vi "Main_Andor_Multi_SI_ver1.vi"() -> ()   [LabVIEW 2014]
doc: "This is the main user interface of the Raman spectroscopy system."
uses:
  <userlib>/atmcd64d.llb/AcquisitionMode_mode typedef.ctl
  <userlib>/atmcd64d.llb/ReadMode_mode typedef.ctl
  <userlib>/atmcd64d.llb/Shutter_mode typedef.ctl
  <userlib>/atmcd64d.llb/Shutter_type typedef.ctl
  <userlib>/atmcd64d.llb/TriggerMode_mode typedef.ctl
  TypeDef/GalvoInput.ctl
  <userlib>/atmcd64d.llb/Error Code Enum typedef.ctl
  TypeDef/States.ctl
panel:
  in  "Tab Control":enum32{"Main", "Andor", "Galvo"}(tab)
  in  "Pause":bool
  in  "Scan Range":T1={"Ver_V/H"=0.35, "Hor_V/W"=0.35, "Ver_r"=5.0, "Hor_r"=5.0}
  in  "Scan Resolusion":T2={"Ver_V"=0.35, "Hor_H"=0.35, "Ver_Pix"=214.0, "Hor_Pix"=200.0}
  in  "Galvo Center":bool
  out "Galvo":bool
  out "Spot Y":dbl
  out "Spot X":dbl
  in  "Quit":bool
  out "Initialization finished":bool
  in  "Galvo Stop":bool
  in  "Galvo Scan":bool
  out "Andor":bool
  out "CurrentFrame":i32
  in  "Set":bool
  in  "AndorSnap":bool
  out "SaveStatus":bool
  in  "FilePath":string="C:\\Users\\light\\Desktop\\Data"
  in  "Exit":bool
  out "ShutDown":cluster{"CoolOff":bool, "ShutDown":bool}
  in  "Mode":T8={"AcqMode"=enum."Single Scan", "ReadMode"=enum."Single-Track", "ShutterMode"=enum."Auto", "GateMode"=enum."TTL High", "TriggerMode"=enum."Internal"}
  in  "AcqSet":T9={"openingtime"=0, "closingtime/ms"=0, "ExposureTime/s"=0.1, "AccumCycTime"=0.0, "AccumCycNum"=1, "KineticNum"=1, "KineticTime"=0.0} {"KineticTime" format="%.5f"; "AccumCycNum" format="%.5f"; "AccumCycTime" format="%.5f"; "ExposureTime/s" format="%.5f"; "closingtime/ms" format="%.2f"; "openingtime" format="%.2f"}
  out "Timing":T10 {"kinetic" format="%.7f"; "accumulate" format="%.7f"; "exposure" format="%.7f"}
  out "SetOut":T11
  in  "MultiTrack":cluster{"StartRow":i32, "EndRow":i32}={"StartRow"=131, "EndRow"=143}
  out "SetStatus":bool
  out "CurrentTemp":i32
  out "DevInit":bool
  out "DevSize":cluster{"xpixels":i32, "ypixels":i32}
  out "HardWVersion":T12
  out "SoftWVersion":T13
  out "Speeds":T14
  in  "TargetTemp":i32
  out "CoolerON":T15
  out "GetStatus":T16
  in  "YOffset":dbl=8.2 caption="Offset"
  in  "XOffset":dbl=4.0 caption="Offset"
  out "Sample Rate":dbl=1000.0 format="%0.2f"
  out "Waveform Graph":waveform(dbl)[](graph)=[{"t0"=timestamp(0 s since 1904-01-01), "dt"=0.001, "Y"=[]}]
  in  "ZOffset":dbl caption="Offset"
  in  "Galvo":T17={"Sample Rate"=1000.0, "Sample Clock Source"="OnboardClock", "Max Voltage"=10.0, "Min Voltage"=-10.0, "Physical Channel(s)"="Dev1/ao0,Dev1/ao1,Dev1/ao3"}
  # "Objective: CFI Plan Fluor ELWD 60x (1.27 NA) \nThe depth of field: 1.78 um\nPixel Size: 0.0877um/px"
  # "Kinetics->SignleTrack"
  # "Galvo Control"
  # "50Hz->1s"
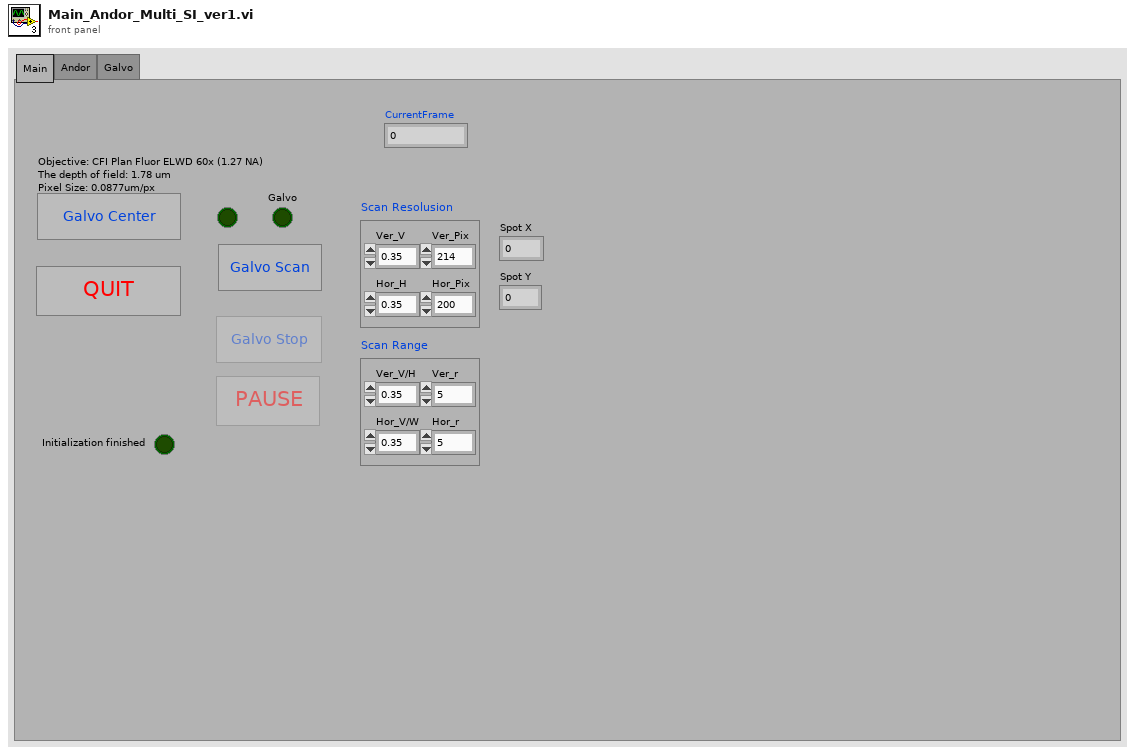
[diagram p1: front panel]
types:
  T1 = cluster{"Ver_V/H":dbl, "Hor_V/W":dbl, "Ver_r":dbl, "Hor_r":dbl}
  T2 = cluster{"Ver_V":dbl, "Hor_H":dbl, "Ver_Pix":dbl, "Hor_Pix":dbl}
  T3 = typedef "AcquisitionMode_mode typedef.ctl" = enum16{"Reserved (0)", "Single Scan", "Accumulate", "Kinetics", "Fast Kinetics", "Run Till Abort", "Reserved (6)", "Reserved (7)", "Reserved (8)", "Time Delayed Integration"}
  T4 = typedef "ReadMode_mode typedef.ctl" = enum16{"Full Vertical Binning", "Multi-Track", "Random-Track", "Single-Track", "Image"}
  T5 = typedef "Shutter_mode typedef.ctl" = enum16{"Auto", "Open", "Close", "N/A (3)", "Open FVB Series", "Open Any Series"}
  T6 = typedef "Shutter_type typedef.ctl" = enum16{"TTL Low", "TTL High"}
  T7 = typedef "TriggerMode_mode typedef.ctl" = enum16{"Internal", "External", "N/A (2)", "N/A (3)", "N/A (4)", "N/A (5)", "External Start", "External Exposure (Bulb)", "N/A (8)", "External FVB EM", "Software", "N/A (11)", "External Charge Shifting"}
  T8 = cluster{"AcqMode":T3, "ReadMode":T4, "ShutterMode":T5, "GateMode":T6, "TriggerMode":T7}
  T9 = cluster{"openingtime":i32, "closingtime/ms":i32, "ExposureTime/s":sgl, "AccumCycTime":sgl, "AccumCycNum":i32, "KineticNum":i32, "KineticTime":sgl}
  T10 = cluster{"exposure":sgl, "accumulate":sgl, "kinetic":sgl}
  T11 = cluster{"Height":i32, "Width":i32, "bottom":i32, "gap":i32}
  T12 = cluster{"PCB":u32, "Flex":u32, "dummy1":u32, "dummy2":u32, "dummy3":u32, "dummy4":u32}
  T13 = cluster{"eprom":u32, "cofFile":u32, "vxdRev":u32, "vxdVer":u32, "dllRev":u32, "dllVer":u32}
  T14 = cluster{"NVS":i32, "VS":i32, "NHS":dbl, "HS":i32}
  T15 = cluster{"SetTemp":bool, "CoolerOn":bool, "Stablized":bool}
  T16 = cluster{"GetDetector":bool, "GetHardVer":bool, "GetNVS":bool, "GetVS":bool, "GetSotfVer":bool, "GetNHS":bool, "GetHS":bool}
  T17 = typedef "GalvoInput.ctl" = cluster{"Sample Rate":dbl, "Sample Clock Source":tag, "Max Voltage":dbl, "Min Voltage":dbl, "Physical Channel(s)":tag}
  T18 = typedef "States.ctl" = enum16{"Initialize", "CMOS live", "Shut down"}
  T19 = enum8{"Enabled", "Disabled", "Disabled and Grayed Out"}
  T20 = typedef "Error Code Enum typedef.ctl" = enum32{"N/A (0)", "DRV_ERROR_CODES", "DRV_SUCCESS", "DRV_VXDNOTINSTALLED", "DRV_ERROR_SCAN", "DRV_ERROR_CHECK_SUM", "DRV_ERROR_FILELOAD", "DRV_UNKNOWN_FUNC", "DRV_ERROR_VXD_INIT", "DRV_ERROR_ADDRESS", "DRV_ERROR_PAGELOCK", "DRV_ERROR_PAGEUNLOCK", "DRV_ERROR_BOARDTEST", "DRV_ERROR_ACK", "DRV_ERROR_UP_FIFO", "DRV_ERROR_PATTERN", "N/A (16)", "DRV_ACQUISITION_ERRORS", "DRV_ACQ_BUFFER", "DRV_ACQ_DOWNFIFO_FULL", "DRV_PROC_UNKONWN_INSTRUCTION", "DRV_ILLEGAL_OP_CODE", "DRV_KINETIC_TIME_NOT_MET", "DRV_ACCUM_TIME_NOT_MET", "DRV_NO_NEW_DATA", "N/A (25)", "DRV_SPOOLERROR", "N/A (27)", "N/A (28)", "N/A (29)", "N/A (30)", "N/A (31)", "N/A (32)", "DRV_TEMPERATURE_CODES", "DRV_TEMPERATURE_OFF", "DRV_TEMPERATURE_NOT_STABILIZED", "DRV_TEMPERATURE_STABILIZED", "DRV_TEMPERATURE_NOT_REACHED", "DRV_TEMPERATURE_OUT_RANGE", "DRV_TEMPERATURE_NOT_SUPPORTED", "DRV_TEMPERATURE_DRIFT", "N/A (41)", "N/A (42)", "N/A (43)", "N/A (44)", "N/A (45)", "N/A (46)", "N/A (47)", "N/A (48)", "DRV_GENERAL_ERRORS", "DRV_INVALID_AUX", "DRV_COF_NOTLOADED", "DRV_FPGAPROG", "DRV_FLEXERROR", "DRV_GPIBERROR", "N/A (55)", "N/A (56)", "N/A (57)", "N/A (58)", "N/A (59)", "N/A (60)", "N/A (61)", "N/A (62)", "N/A (63)", "DRV_DATATYPE", "DRV_DRIVER_ERRORS", "DRV_P1INVALID", "DRV_P2INVALID", "DRV_P3INVALID", "DRV_P4INVALID", "DRV_INIERROR", "DRV_COFERROR", "DRV_ACQUIRING", "DRV_IDLE", "DRV_TEMPCYCLE", "DRV_NOT_INITIALIZED", "DRV_P5INVALID", "DRV_P6INVALID", "DRV_INVALID_MODE", "DRV_INVALID_FILTER", "DRV_I2CERRORS", "DRV_I2CDEVNOTFOUND", "DRV_I2CTIMEOUT", "DRV_P7INVALID", "N/A (84)", "N/A (85)", "N/A (86)", "N/A (87)", "N/A (88)", "N/A (89)", "DRV_IOCERROR", "DRV_VRMVERSIONERROR"}
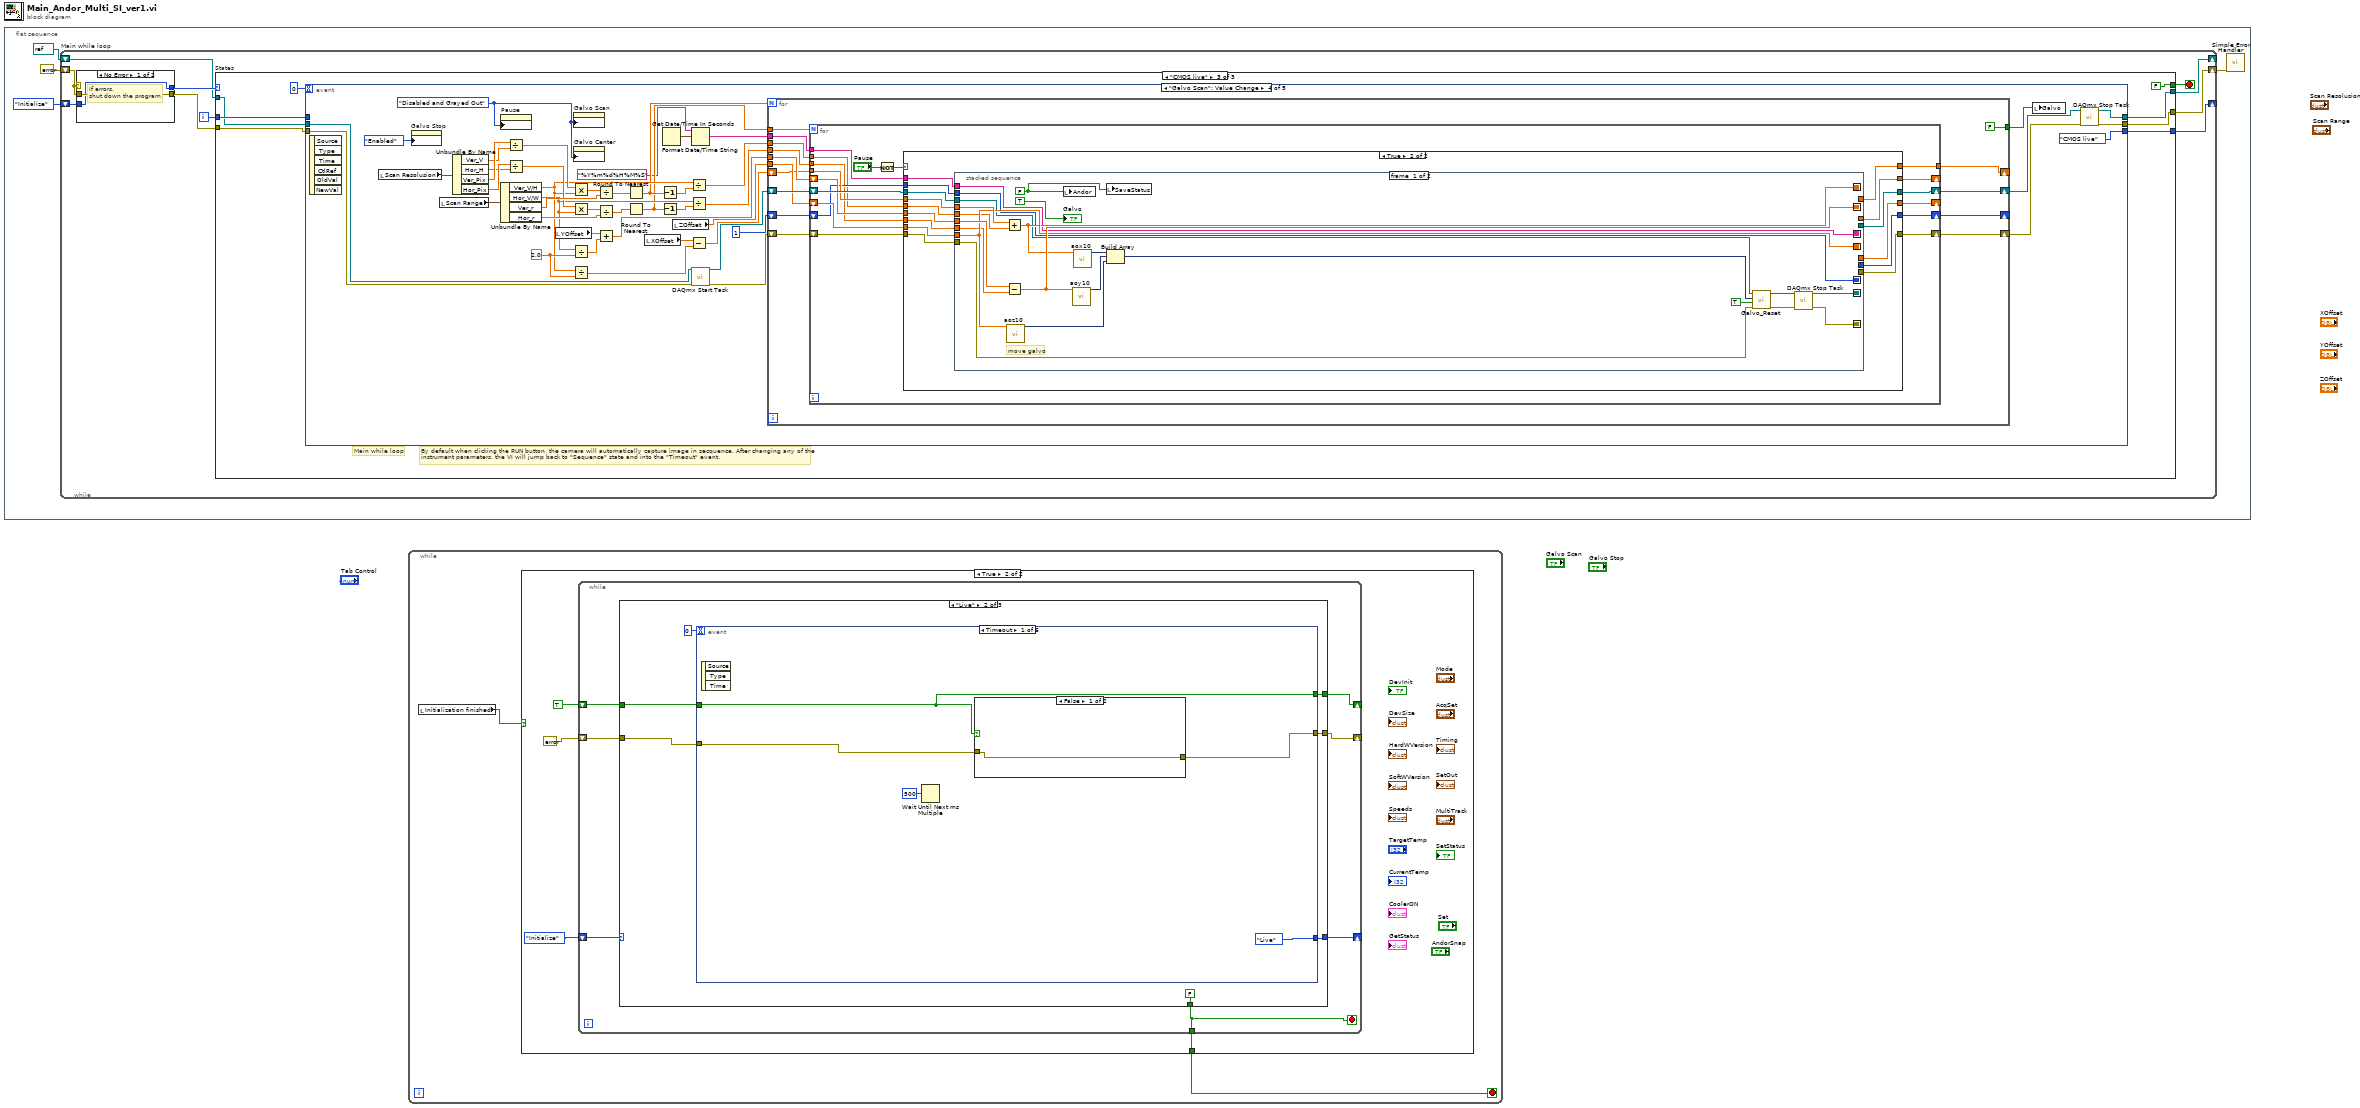
[diagram p0: block diagram]
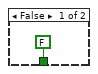
[diagram p2: hidden frame]
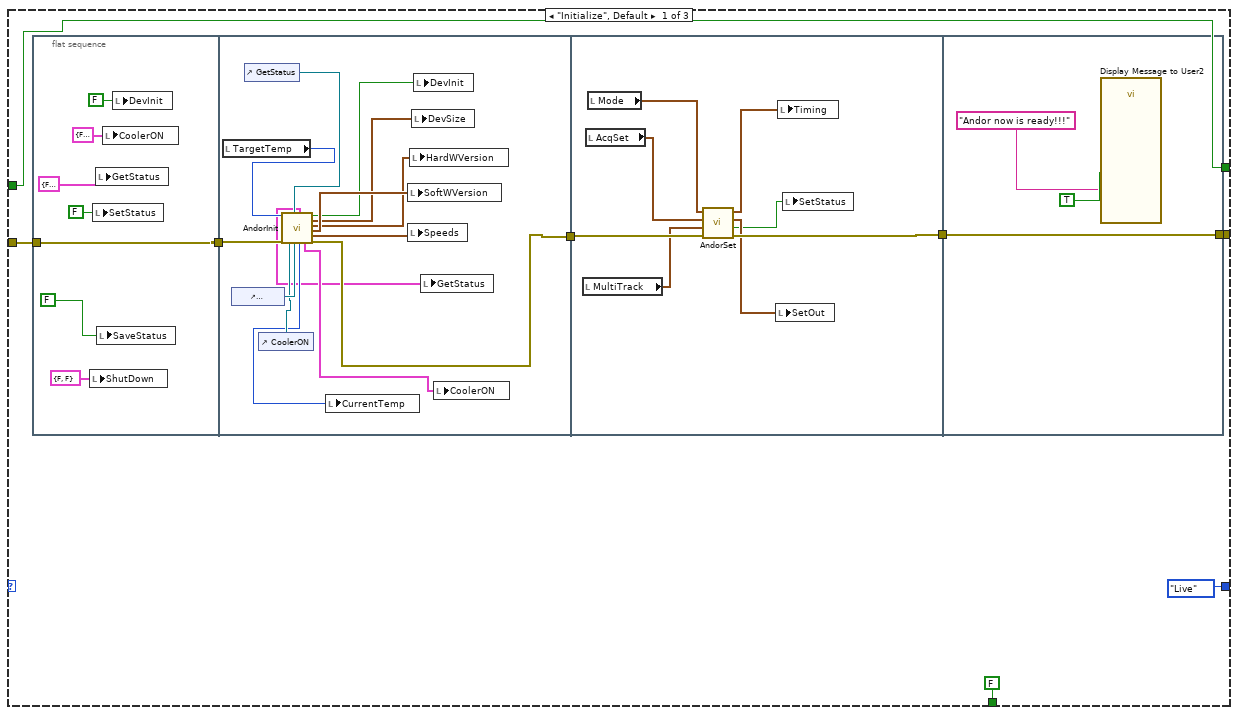
[diagram p3: hidden frame]
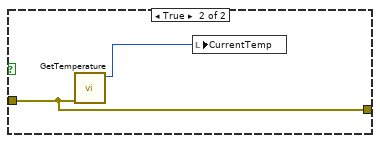
[diagram p4: hidden frame]
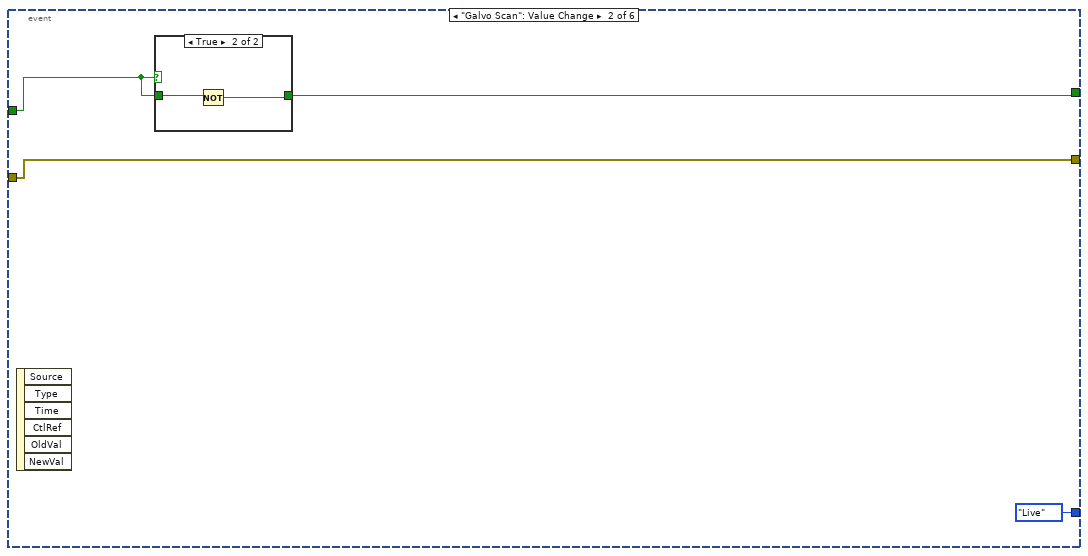
[diagram p5: hidden frame]
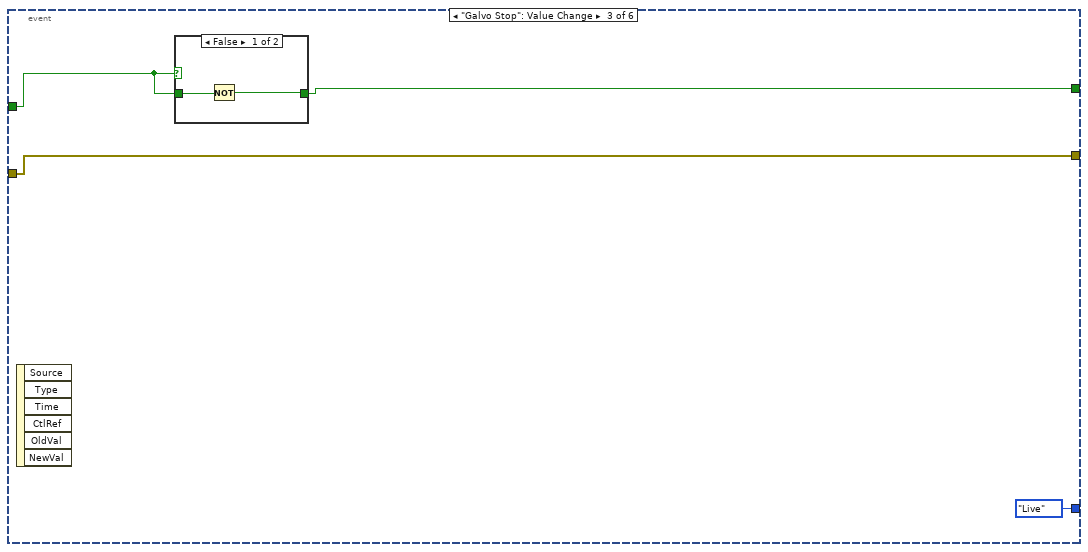
[diagram p7: hidden frame]
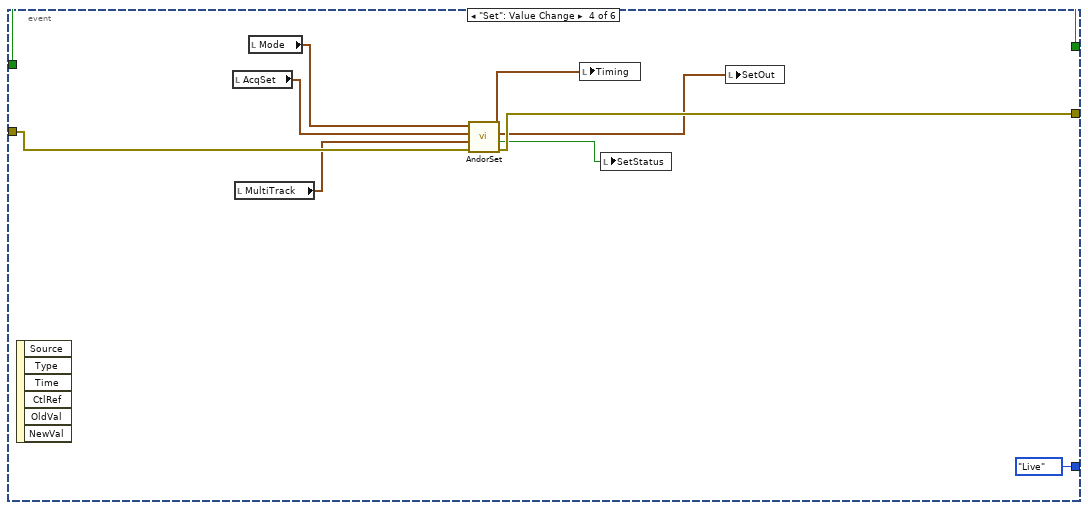
[diagram p9: hidden frame]
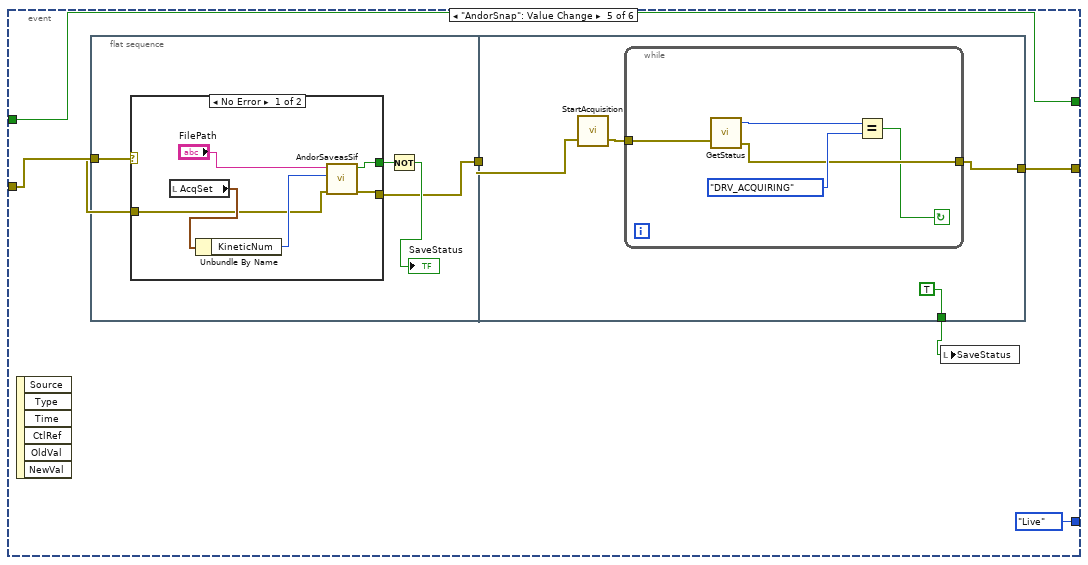
[diagram p10: hidden frame]
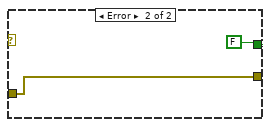
[diagram p11: hidden frame]
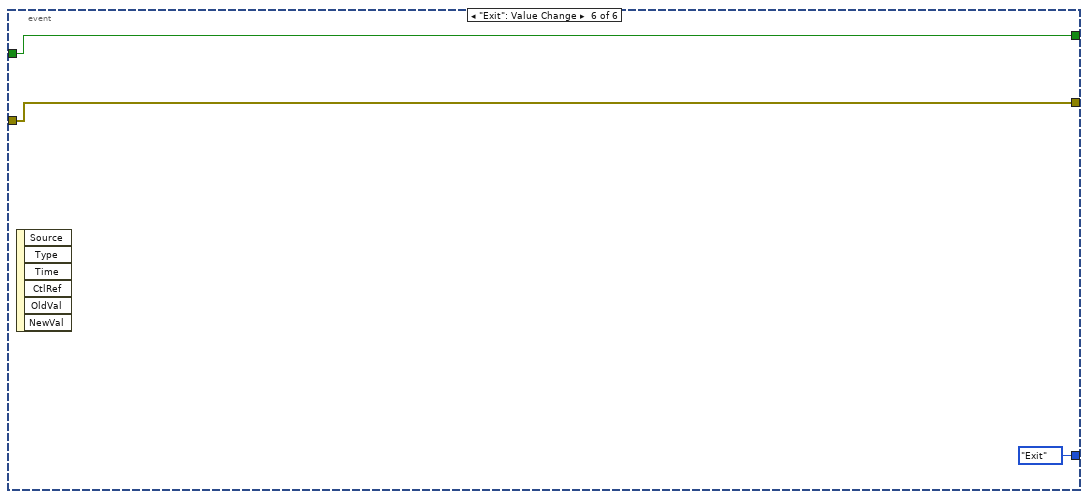
[diagram p12: hidden frame]
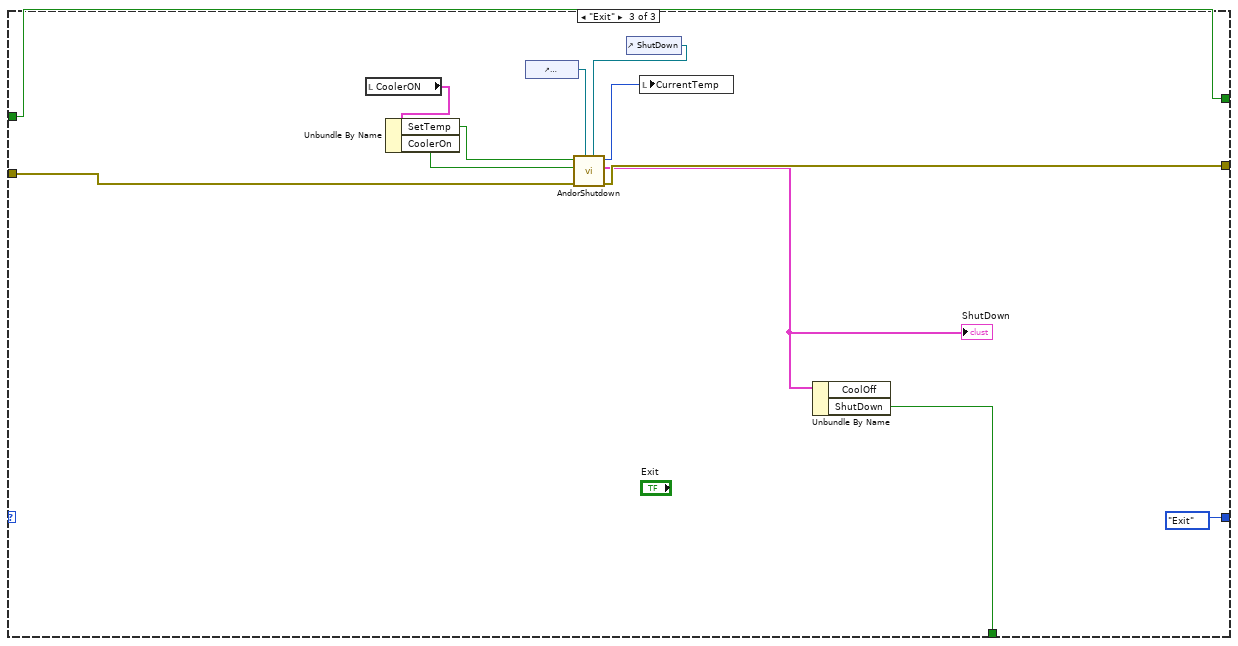
[diagram p13: hidden frame]
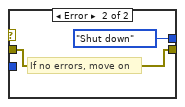
[diagram p14: hidden frame]
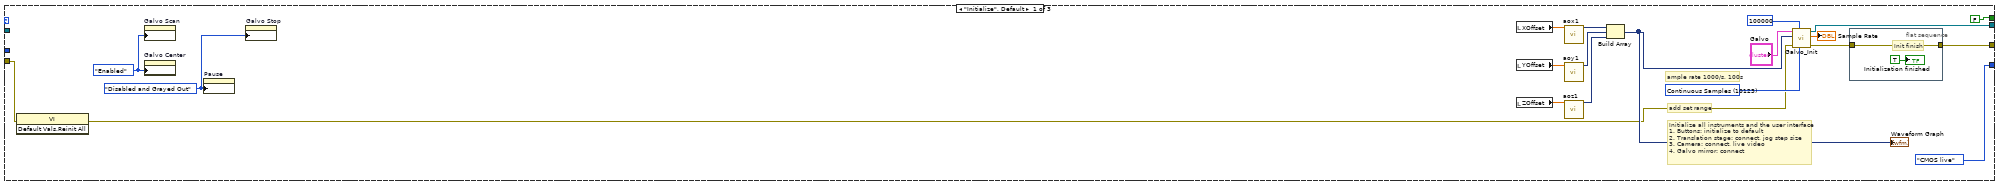
[diagram p15: hidden frame]
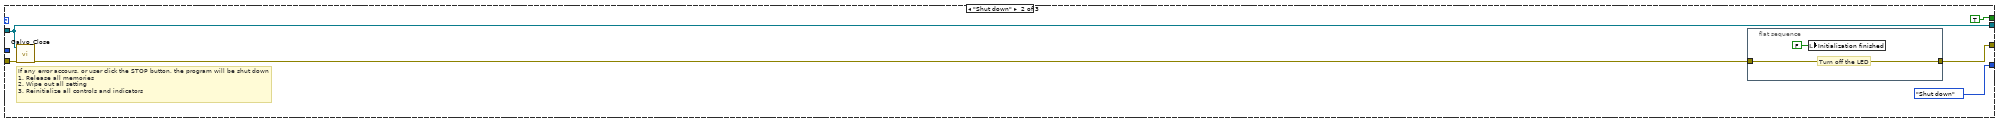
[diagram p16: hidden frame]
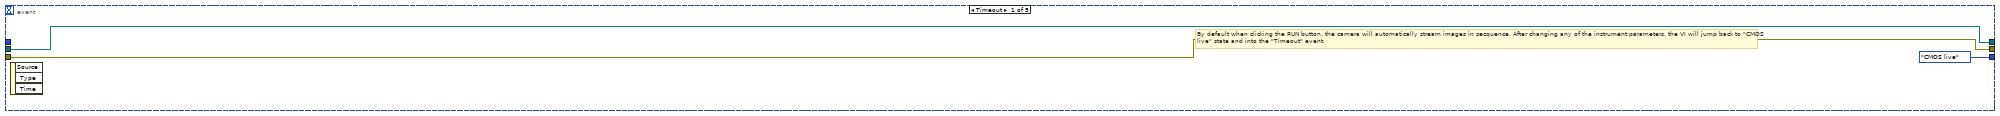
[diagram p17: hidden frame]
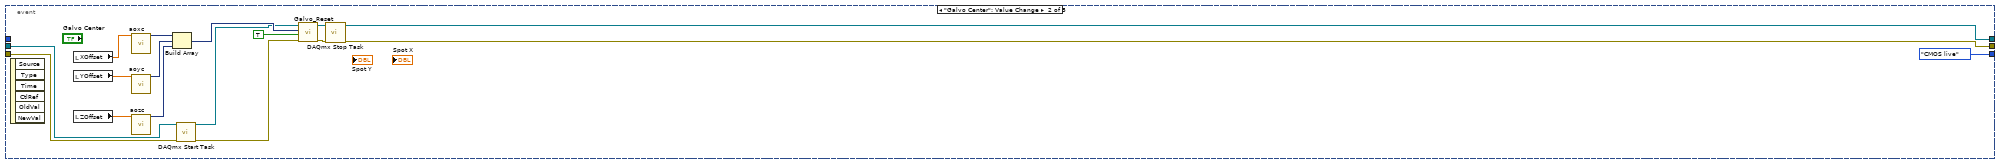
[diagram p18: hidden frame]
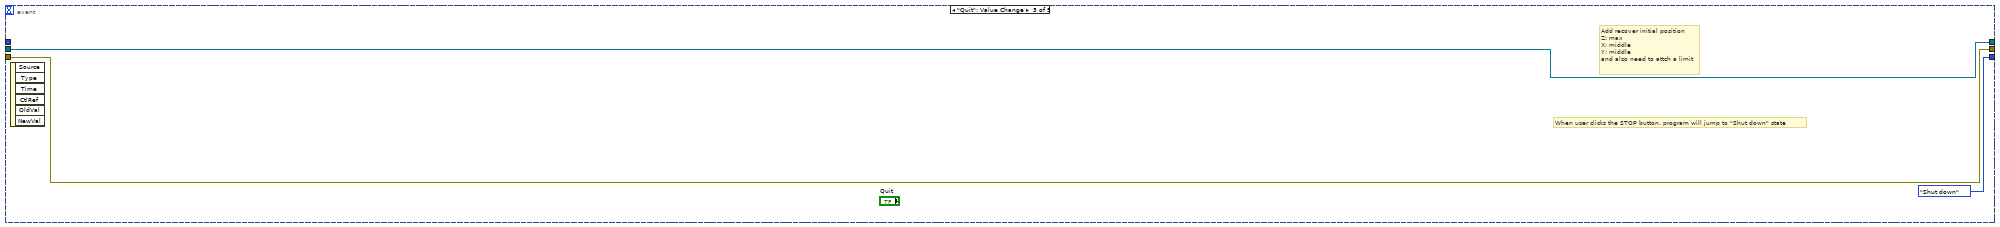
[diagram p19: hidden frame]
diagram:
  n1 = flat-sequence {
    frame #0 {
      n2 = while "Main while loop" {
        shift-right: [w9] -> _
        shift-left: States."Initialize" -> [w14]
        shift-right: [w12] -> w2
        shift-left: errorcluster {"status"=FALSE, "code"=0, "source"=""} ("error out") -> [w8]
        shift-right: [w6] -> _
        shift-left: refnum<k21> refnum ("task out") -> [w5]
        i -> [w7]
        stop <- w10 stop-if-true
        n3 = case shown="No Error" w8 {
          tunnel: w8 -> [w16 w18]
          tunnel: [w16 w18] -> w11
          tunnel: w14 -> [w15 _]
          tunnel: [w15 States."Shut down"] -> w13
          frame No Error {
            # "If errors,\nshut down the program"
          }
          frame Error {
            # "If no errors, move on"
          }
        }
        n4 = case "States" shown="\"CMOS live\"" w13 {
          tunnel: [w36 w41 w54] -> w12
          tunnel: w11 -> [w37 w42 w55]
          tunnel: [FALSE TRUE FALSE] -> w10
          tunnel: [States."CMOS live" States."Shut down" w56] -> w9
          tunnel: w7 -> [_ _ w52]
          tunnel: [w33 w44 w50] -> w6
          tunnel: w5 -> [_ w44 w51]
          frame "Initialize", Default {
            w19 = T19."Disabled and Grayed Out" ("Disabled")
            w22 = T19."Enabled" ("Disabled")
            w28 = 10123 items=["Finite Samples"=10178, "Continuous Samples"=10123, "Hardware Timed Single Point"=12522] ("Sample Mode")
            # "ample rate 1000/s, 100s"
            # "add set range"
            # "Initialize all instruments and the user interface\n1. Buttons: initialize to default\n2. Translation stage: connect, jog step size\n3. Camera: connect, live video\n4. Galvo mirror: connect"
            n5 = invoke class="VI" method="Default Vals.Reinit All"(error in=w37) -> (error out=w21:errorcluster)  [unwired: 2 in, 2 out]
            n6 = property on="Galvo Scan" class="Bool"("DisabledEnum"=w22) -> ()  [unwired: 2 in, 2 out]
            n7 = property on="Galvo Center" class="Bool"("DisabledEnum"=w22) -> ()  [unwired: 2 in, 2 out]
            n8 = property on="Pause" class="Bool"("DisabledEnum"=w19) -> ()  [unwired: 2 in, 2 out]
            n9 = property on="Galvo Stop" class="Bool"("DisabledEnum"=w19) -> ()  [unwired: 2 in, 2 out]
            n10 = local read "XOffset"() -> (w25:dbl)
            n11 = local read "YOffset"() -> (w24:dbl)
            n12 = local read "ZOffset"() -> (w23:dbl)
            n13 = call "aox1"("Offset"=w25) -> ("DC"=w27:dynamicdata)  [unwired: 13 in, 1 out]
            n14 = call "aoy1"("Offset"=w24) -> ("DC"=w26:dynamicdata)  [unwired: 13 in, 1 out]
            n15 = call "aoz1"("Offset"=w23) -> ("DC"=w31:dynamicdata)  [unwired: 13 in, 1 out]
            n16 = Build Array(w27, w26, w31) -> (w30:dynamicdata[])
            "Waveform Graph" <- w30
            n17 = call "Galvo_Init.vi"("Sample Mode"=w28, "samples per channel"=100000, "error in"=w21, "Signal array"=w30, "Galvo_Input"="Galvo") -> ("error out"=w32:errorcluster, "Actual Sample Rate"=→"Sample Rate":dbl, "task out"=w33:refnum<k21>)  [unwired: 4 in]
            n18 = flat-sequence {
              tunnel: w32 -> [w40]
              tunnel: [w40] -> w36
              frame #0 {
                # "Init finish"
                "Initialization finished" <- TRUE ("Initialization finished")
              }
            }
          }
          frame "Shut down" {
            # "If any error accours, or user click the STOP button, the program will be shut down\n1. Release all memories\n2. Wipe out all setting\n3. Reinitialize all controls and indicators"
            n19 = call "Galvo_Close.vi"("error in"=w42, "task/channels in"=w44) -> ("error out"=w43:errorcluster)  [unwired: 9 in]
            n20 = flat-sequence {
              tunnel: w43 -> [w47]
              tunnel: [w47] -> w41
              frame #0 {
                # "Turn off the LED"
                n21 = local write "Initialization finished"(FALSE ("Initialization finished")) -> ()
              }
            }
          }
          frame "CMOS live" {
            # "Main while loop"
            # "By default when clicking the RUN button, the camera will automatically capture image in secquence. After changing any of the \ninstrument parameters, the VI will jump back to \"Sequence\" state and into the \"Timeout\" event."
            n22 = event shown="[3] \"Galvo Scan\": Value Change" {
              selector: _ -> [_ _ _ _ _]
              dyn-events: _ -> [_ _ _ _ _]
              timeout: 0 -> [_ _ _ _ _]
              tunnel: [States."CMOS live" States."CMOS live" States."Shut down" States."CMOS live" States."CMOS live"] -> w56
              tunnel: w55 -> [w57 w68 w78 w82 w254]
              tunnel: [w57 w62 w78 w109 w254] -> w54
              tunnel: w52 -> [_ _ _ _ _]
              tunnel: [w59 w63 w77 w108 w256] -> w50
              tunnel: w51 -> [w59 w70 w77 w124 w256]
              event Timeout {
                # "By default when clicking the RUN button, the camera will automatically stream images in secquence. After changing any of the instrument parameters, the VI will jump back to \"CMOS live\" state and into the \"Timeout\" event."
                n23 = event-data() -> ()  [unwired: 1 in, 3 out]
              }
              event "Galvo Center": Value Change {
                n24 = event-data() -> ()  [unwired: 1 in, 6 out]
                n25 = local read "XOffset"() -> (w61:dbl)
                n26 = local read "YOffset"() -> (w60:dbl)
                n27 = local read "ZOffset"() -> (w74:dbl)
                n28 = call "aoxc"("Offset"=w61) -> ("DC"=w72:dynamicdata)  [unwired: 13 in, 1 out]
                n29 = call "aoyc"("Offset"=w60) -> ("DC"=w71:dynamicdata)  [unwired: 13 in, 1 out]
                n30 = call "aozc"("Offset"=w74) -> ("DC"=w75:dynamicdata)  [unwired: 13 in, 1 out]
                n31 = Build Array(w72, w71, w75) -> (w73:dynamicdata[])
                n32 = call <vilib>:"DAQmx Start Task.vi"("task/channels in"=w70, "error in"=w68) -> ("task out"=w69:refnum<k21>, "error out"=w67:errorcluster)  [unwired: 12 in]
                n33 = call "Galvo_Reset.vi"("error in"=w67, "auto start"=TRUE, "Signal array"=w73, "task/channels in"=w69) -> ("error out"=w64:errorcluster, "task out"=w65:refnum<k21>)  [unwired: 6 in]
                n34 = call <vilib>:"DAQmx Stop Task.vi"("task/channels in"=w65, "error in"=w64) -> ("task out"=w63:refnum<k21>, "error out"=w62:errorcluster)  [unwired: 12 in]
              }
              event "Quit": Value Change {
                # "Add recover initial position\nZ: max\nX: middle\nY: middle\nand also need to attch a limit"
                # "When user clicks the STOP button, program will jump to \"Shut down\" state"
                n35 = event-data() -> ()  [unwired: 1 in, 6 out]
              }
              event "Galvo Scan": Value Change {
                w107 = 2.0 ("y")
                w80 = T19."Disabled and Grayed Out" ("Disabled")
                n36 = event-data() -> ()  [unwired: 1 in, 6 out]
                n37 = local read "Scan Resolusion"() -> (w123:T2)
                n38 = property on="Galvo Stop" class="Bool"("DisabledEnum"=T19."Enabled" ("Disabled")) -> ()  [unwired: 2 in, 2 out]
                n39 = local read "Scan Range"() -> (w120:T1)
                n40 = Unbundle By Name(w123) -> ("Ver_V"=w121:dbl, "Hor_H"=w94:dbl, "Ver_Pix"=w122:dbl, "Hor_Pix"=w95:dbl)
                n41 = property on="Pause" class="Bool"("DisabledEnum"=w80) -> ()  [unwired: 2 in, 2 out]
                n42 = Unbundle By Name(w120) -> ("Ver_V/H"=w93:dbl, "Hor_V/W"=w92:dbl, "Ver_r"=w118:dbl, "Hor_r"=w116:dbl)
                n43 = Divide(x=w122, y=w121) -> (x/y=w99:dbl)
                n44 = Divide(x=w95, y=w94) -> (x/y=w98:dbl)
                n45 = local read "YOffset"() -> (w104:dbl)
                n46 = Multiply(x=w99, y=w93) -> (x*y=w119:dbl)
                n47 = Multiply(x=w98, y=w92) -> (x*y=w117:dbl)
                n48 = Divide(x=w92, y=w107) -> (x/y=w103:dbl)
                n49 = Divide(x=w93, y=w107) -> (x/y=w105:dbl)
                n50 = property on="Galvo Scan" class="Bool"("DisabledEnum"=w80) -> ()  [unwired: 2 in, 2 out]
                n51 = property on="Galvo Center" class="Bool"("DisabledEnum"=w80) -> ()  [unwired: 2 in, 2 out]
                n52 = Divide(x=w119, y=w118) -> (x/y=w115:dbl)
                n53 = Divide(x=w117, y=w116) -> (x/y=w96:dbl)
                n54 = Add(x=w104, y=w103) -> (x+y=w101:dbl)
                n55 = Round To Nearest(number=w115) -> (nearest integer value=w91:dbl)
                n56 = Round To Nearest(number=w96) -> (nearest integer value=w89:dbl)
                n57 = local read "XOffset"() -> (w106:dbl)
                n58 = Decrement(x=w91) -> (x-1=w90:dbl)
                n59 = Decrement(x=w89) -> (x-1=w88:dbl)
                n60 = Get Date/Time In Seconds() -> (seconds since 1Jan1904=w85:timestamp)
                n61 = local read "ZOffset"() -> (w100:dbl)
                n62 = Divide(x=w93, y=w90) -> (x/y=w87:dbl)
                n63 = Divide(x=w92, y=w88) -> (x/y=w86:dbl)
                n64 = Subtract(x=w106, y=w105) -> (x-y=w102:dbl)
                n65 = Format Date/Time String(time format string (%c)="%Y%m%d%H%M%S", seconds (now)=w85) -> (date/time string=w83:string)  [unwired: 1 in]
                n66 = call <vilib>:"DAQmx Start Task.vi"("task/channels in"=w124, "error in"=w82) -> ("task out"=w112:refnum<k21>, "error out"=w114:errorcluster)  [unwired: 12 in]
                n67 = for {
                  N: w91 -> [_]
                  tunnel: [FALSE ("Galvo")] -> w113
                  shift-right: [w139] -> w110
                  shift-left: w114 -> [w138]
                  shift-right: [w132] -> _
                  shift-left: w102 -> [w133]
                  shift-right: [w136] -> w111
                  shift-left: w112 -> [w137]
                  tunnel: w101 -> [w135]
                  tunnel: w100 -> [w134]
                  shift-right: [w130] -> _
                  shift-left: 1 -> [w131]
                  tunnel: w89 -> [w129]
                  tunnel: w87 -> [w128]
                  tunnel: w86 -> [w127]
                  tunnel: w83 -> [w126]
                  n68 = for {
                    N: w129 -> [_]
                    shift-right: [w145] -> w139
                    shift-left: w138 -> [w157]
                    shift-right: [w143] -> _
                    shift-left: w135 -> [w154]
                    shift-right: [w144] -> _
                    shift-left: w134 -> [w153]
                    shift-right: [w146] -> w136
                    shift-left: w137 -> [w156]
                    tunnel: w133 -> [w155]
                    tunnel: [w142] -> w132
                    shift-right: [w141] -> w130
                    shift-left: w131 -> [w152]
                    tunnel: w128 -> [w151]
                    tunnel: w127 -> [w150]
                    tunnel: w126 -> [w149]
                    n69 = Not(x="Pause") -> (.not. x?=w147:bool)
                    n70 = case shown="True" w147 {
                      tunnel: w157 -> [w160 w178]
                      tunnel: w156 -> [w159 w177]
                      tunnel: w155 -> [w161 w176]
                      tunnel: w154 -> [w162 w175]
                      tunnel: w153 -> [w163 w174]
                      tunnel: [w162 w173] -> w143
                      tunnel: [w163 w166] -> w144
                      tunnel: [w161 w172] -> w142
                      tunnel: w152 -> [w158 w171]
                      tunnel: w151 -> [_ w170]
                      tunnel: w150 -> [_ w169]
                      tunnel: w149 -> [_ w168]
                      tunnel: [w160 w167] -> w145
                      tunnel: [w159 w165] -> w146
                      tunnel: [w158 w164] -> w141
                      frame False {
                      }
                      frame True {
                        n71 = stacked-sequence {
                          seq-local: [w185 _] -> [_ w205]
                          seq-local: [w191 _] -> [_ w208]
                          seq-local: [w190 _] -> [_ w207]
                          seq-local: [w189 _] -> [_ w206]
                          seq-local: [w183 _] -> [_ w213]
                          seq-local: [w182 _] -> [_ w204]
                          seq-local: [w179 _] -> [_ w203]
                          tunnel: w178 -> [w192 _]
                          tunnel: w177 -> [w181 _]
                          tunnel: w176 -> [w194 _]
                          tunnel: w175 -> [w193 _]
                          tunnel: w174 -> [w190 _]
                          tunnel: w171 -> [w183 _]
                          tunnel: w170 -> [w188 _]
                          tunnel: w169 -> [w187 _]
                          tunnel: w168 -> [w182 _]
                          tunnel: [_ w208] -> w173
                          tunnel: [_ w207] -> w166
                          tunnel: [_ w206] -> w172
                          tunnel: [_ w211] -> w164
                          tunnel: [_ w210] -> w167
                          tunnel: [_ w201] -> w165
                          frame #0 {
                            w197 = FALSE ("SaveStatus")
                            # "move galvo"
                            n72 = Add(x=w194, y=w188) -> (x+y=w189:dbl)
                            n73 = Subtract(x=w193, y=w187) -> (x-y=w191:dbl)
                            n74 = call "aoz10"("Offset"=w190) -> ("DC"=w200:dynamicdata)  [unwired: 13 in, 1 out]
                            n75 = local write "Andor"(w197) -> ()
                            n76 = call "aoy10"("Offset"=w191) -> ("DC"=w198:dynamicdata)  [unwired: 13 in, 1 out]
                            n77 = call "aox10"("Offset"=w189) -> ("DC"=w199:dynamicdata)  [unwired: 13 in, 1 out]
                            n78 = local write "SaveStatus"(w197) -> ()
                            n79 = Build Array(w199, w198, w200) -> (w195:dynamicdata[])
                            n80 = call "Galvo_Reset.vi"("error in"=w192, "auto start"=TRUE, "Signal array"=w195, "task/channels in"=w181) -> ("error out"=w186:errorcluster, "task out"=w180:refnum<k21>)  [unwired: 6 in]
                            n81 = call <vilib>:"DAQmx Stop Task.vi"("task/channels in"=w180, "error in"=w186) -> ("task out"=w179:refnum<k21>, "error out"=w185:errorcluster)  [unwired: 12 in]
                            "Galvo" <- TRUE
                          }
                          frame #1 {
                            n82 = flat-sequence {
                              tunnel: [w221] -> w214
                              tunnel: w213 -> [w219]
                              tunnel: [w218] -> w212
                              tunnel: w205 -> [w217]
                              tunnel: w204 -> [w216]
                              tunnel: w203 -> [w215]
                              tunnel: [w215] -> w202
                              tunnel: [w239] -> w210
                              tunnel: w214 -> [w237]
                              tunnel: w212 -> [w238]
                              tunnel: [w238] -> w211
                              tunnel: [FALSE ("Galvo")] -> w209
                              tunnel: w202 -> [w235]
                              tunnel: [w234] -> w201
                              frame #0 {
                                n83 = case shown="No Error" w217 {
                                tunnel: [w229 w231] -> w221
                                tunnel: [w228 w232] -> w218
                                tunnel: [w227 FALSE ("SaveStatus")] -> w220
                                tunnel: w219 -> [w226 w232]
                                tunnel: w217 -> [w223 w231]
                                tunnel: w216 -> [w222 _]
                                frame No Error {
                                n84 = local read "AcqSet"() -> (w225:T9)
                                n85 = Unbundle By Name(w225) -> ("KineticNum"=w224:i32)
                                n86 = local read "FilePath"() -> (w230:string)
                                n87 = Increment(x=w226) -> (x+1=w228:i32)
                                n88 = call "AndorSaveasSif_Ver2.vi"("Time"=w222, "error in"=w223, "No."=w226, "KinNumber"=w224, "FilePath"=w230) -> ("error out"=w229:errorcluster, "SaveStatus"=w227:bool)  [unwired: 5 in]
                                "CurrentFrame" <- w226
                                }
                                frame Error {
                                }
                                }
                                n89 = local write "SaveStatus"(w220) -> ()
                              }
                              frame #1 {
                                n90 = flat-sequence {
                                tunnel: [w247] -> w241
                                tunnel: [TRUE] -> w240
                                tunnel: w237 -> [w245]
                                tunnel: [w243] -> w234
                                tunnel: w235 -> [w242]
                                frame #0 {
                                n91 = call <vilib>:"DAQmx Start Task.vi"("task/channels in"=w242, "error in"=w245) -> ("task out"=w243:refnum<k21>, "error out"=w244:errorcluster)  [unwired: 12 in]
                                n92 = call <userlib>:"StartAcquisition.vi"("error in (no error)"=w244) -> ("error out"=w247:errorcluster)  [unwired: 1 in, 1 out]
                                }
                                }
                                n93 = local write "Andor"(w240) -> ()
                                n94 = while {
                                tunnel: w241 -> [w252]
                                tunnel: [w249] -> w239
                                stop <- w248 continue-if-true
                                n95 = call <userlib>:"GetStatus.vi"("error in (no error)"=w252) -> ("error out"=w249:errorcluster, "status"=w251:T20)  [unwired: 2 in, 1 out]
                                n96 = Equal?(x=Error_Code_Enum_typedef."DRV_ACQUIRING" ("y"), y=w251) -> (x = y?=w248:bool)
                                "Andor" <- w248
                                }
                              }
                            }
                            n97 = local write "Galvo"(w209) -> ()
                          }
                        }
                      }
                    }
                  }
                }
                n98 = local write "Galvo"(w113) -> ()
                n99 = call <vilib>:"DAQmx Stop Task.vi"("task/channels in"=w111, "error in"=w110) -> ("task out"=w108:refnum<k21>, "error out"=w109:errorcluster)  [unwired: 12 in]
              }
              event "Galvo Stop": Value Change {
                w255 = T19."Enabled" ("Disabled")
                n100 = event-data() -> ()  [unwired: 1 in, 6 out]
                n101 = property on="Galvo Scan" class="Bool"("DisabledEnum"=w255) -> ()  [unwired: 2 in, 2 out]
                n102 = property on="Galvo Center" class="Bool"("DisabledEnum"=w255) -> ()  [unwired: 2 in, 2 out]
                n103 = property on="Pause" class="Bool"("DisabledEnum"=T19."Disabled and Grayed Out" ("Disabled")) -> ()  [unwired: 2 in, 2 out]
              }
            }
          }
        }
      }
      n104 = call <vilib>:"Simple Error Handler.vi"("error in (no error)"=w2) -> ()  [unwired: 4 in, 5 out]
    }
  }
  n105 = while {
    stop <- w258 stop-if-true
    n106 = local read "Initialization finished"() -> (w259:bool)
    n107 = case shown="True" w259 {
      tunnel: [FALSE ("ShutDown") w262] -> w258
      frame False {
      }
      frame True {
        n108 = while {
          shift-right: [w270] -> _
          shift-left: enum16{"Initialize", "Live", "Exit"}."Initialize" -> [w271]
          shift-right: [w268] -> _
          shift-left: errorcluster {"status"=FALSE, "code"=0, "source"=""} ("error in") -> [w269]
          tunnel: [w267] -> w262
          shift-right: [w265] -> _
          shift-left: TRUE -> [w266]
          stop <- w267 stop-if-true
          n109 = case shown="\"Live\"" w271 {
            tunnel: [enum16{"Initialize", "Live", "Exit"}."Live" w318 enum16{"Initialize", "Live", "Exit"}."Exit"] -> w270
            tunnel: w269 -> [w277 w317 w391]
            tunnel: [w274 w316 w390] -> w268
            tunnel: [FALSE ("ShutDown") FALSE ("ShutDown") w382] -> w267
            tunnel: w266 -> [w272 w313 w381]
            tunnel: [w272 w312 w381] -> w265
            frame "Initialize", Default {
              n110 = flat-sequence {
                tunnel: [w286] -> w278
                tunnel: w277 -> [w286]
                tunnel: w278 -> [w300]
                tunnel: [w299] -> w276
                tunnel: w276 -> [w308]
                tunnel: [w307] -> w275
                tunnel: w275 -> [w311]
                tunnel: [w311] -> w274
                frame #0 {
                  n111 = local write "ShutDown"(cluster{"CoolOff":bool, "ShutDown":bool} {"CoolOff"=FALSE, "ShutDown"=FALSE} ("ShutDown")) -> ()
                  n112 = local write "SetStatus"(FALSE ("SetStatus")) -> ()
                  n113 = local write "GetStatus"(T16 {"GetDetector"=FALSE, "GetHardVer"=FALSE, "GetNVS"=FALSE, "GetVS"=FALSE, "GetSotfVer"=FALSE, "GetNHS"=FALSE, "GetHS"=FALSE} ("GetStatus")) -> ()
                  n114 = local write "SaveStatus"(FALSE ("Save")) -> ()
                  n115 = local write "CoolerON"(T15 {"SetTemp"=FALSE, "CoolerOn"=FALSE, "Stablized"=FALSE} ("CoolerON")) -> ()
                  n116 = local write "DevInit"(FALSE ("DevInit")) -> ()
                }
                frame #1 {
                  n117 = local read "TargetTemp"() -> (w295:i32)
                  n118 = control-ref of="CurrentTemp"() -> (w297:refnum<vi>)
                  n119 = control-ref of="GetStatus"() -> (w298:refnum<vi>)
                  n120 = control-ref of="CoolerON"() -> (w296:refnum<vi>)
                  n121 = call "AndorInit.vi"("TargetTemp"=w295, "error in"=w300, "CoolerONRef"=w296, "GetStatusRef"=w298, "CurrentTempRef"=w297) -> ("GetStatus"=w287:T16, "CurrentTemp"=w294:i32, "CoolerON"=w293:T15, "DevInit"=w290:bool, "DevSize"=w289:cluster{"xpixels":i32, "ypixels":i32}, "HardWVersion"=w288:T12, "SoftWVersion"=w291:T13, "Speeds"=w292:T14, "error out"=w299:errorcluster)  [unwired: 6 in]
                  n122 = local write "CurrentTemp"(w294) -> ()
                  n123 = local write "SoftWVersion"(w291) -> ()
                  n124 = local write "Speeds"(w292) -> ()
                  n125 = local write "HardWVersion"(w288) -> ()
                  n126 = local write "DevSize"(w289) -> ()
                  n127 = local write "DevInit"(w290) -> ()
                  n128 = local write "GetStatus"(w287) -> ()
                  n129 = local write "CoolerON"(w293) -> ()
                }
                frame #2 {
                  n130 = local read "MultiTrack"() -> (w304:cluster{"StartRow":i32, "EndRow":i32})
                  n131 = local read "AcqSet"() -> (w306:T9)
                  n132 = local read "Mode"() -> (w305:T8)
                  n133 = call "AndorSet.vi"("error in"=w308, "MultiTrack"=w304, "AcqSet"=w306, "Mode"=w305) -> ("error out"=w307:errorcluster, "SetStatus"=w301:bool, "SetOut"=w302:T11, "Timing"=w303:T10)  [unwired: 4 in]
                  n134 = local write "SetOut"(w302) -> ()
                  n135 = local write "Timing"(w303) -> ()
                  n136 = local write "SetStatus"(w301) -> ()
                }
                frame #3 {
                  n137 = call "Display Message to User2"("Enable"=TRUE, "Message"="Andor now is ready!!!") -> ()  [unwired: 8 in, 2 out]
                }
              }
            }
            frame "Live" {
              n138 = event shown="[0] Timeout" {
                selector: _ -> [_ _ _ _ _ _]
                dyn-events: _ -> [_ _ _ _ _ _]
                timeout: 0 -> [_ _ _ _ _ _]
                tunnel: [enum16{"Initialize", "Live", "Exit"}."Live" enum16{"Initialize", "Live", "Exit"}."Live" enum16{"Initialize", "Live", "Exit"}."Live" enum16{"Initialize", "Live", "Exit"}."Live" enum16{"Initialize", "Live", "Exit"}."Live" enum16{"Initialize", "Live", "Exit"}."Exit"] -> w318
                tunnel: w317 -> [w321 w330 w337 w349 w354 w379]
                tunnel: [w320 w330 w337 w348 w352 w379] -> w316
                tunnel: w313 -> [w319 w328 w335 w341 w351 w378]
                tunnel: [w319 w327 w334 w341 w351 w378] -> w312
                event Timeout {
                  n139 = event-data() -> ()  [unwired: 1 in, 3 out]
                  n140 = Wait Until Next ms Multiple(millisecond multiple=u32 500) -> ()  [unwired: 1 out]
                  n141 = case shown="False" w319 {
                    tunnel: w321 -> [w324 w325]
                    tunnel: [w324 w325] -> w320
                    frame False {
                    }
                    frame True {
                      n142 = call <userlib>:"GetTemperature.vi"("error in (no error)"=w325) -> ("temperature"=w326:i32)  [unwired: 3 in, 3 out]
                      n143 = local write "CurrentTemp"(w326) -> ()
                    }
                  }
                }
                event "Galvo Scan": Value Change {
                  n144 = event-data() -> ()  [unwired: 1 in, 6 out]
                  n145 = case shown="True" w328 {
                    tunnel: w328 -> [w331 w333]
                    tunnel: [w331 w332] -> w327
                    frame False {
                    }
                    frame True {
                      n146 = Not(x=w333) -> (.not. x?=w332:bool)
                    }
                  }
                }
                event "Galvo Stop": Value Change {
                  n147 = event-data() -> ()  [unwired: 1 in, 6 out]
                  n148 = case shown="False" w335 {
                    tunnel: w335 -> [w339 w340]
                    tunnel: [w338 w340] -> w334
                    frame False {
                      n149 = Not(x=w339) -> (.not. x?=w338:bool)
                    }
                    frame True {
                    }
                  }
                }
                event "Set": Value Change {
                  n150 = event-data() -> ()  [unwired: 1 in, 6 out]
                  n151 = local read "AcqSet"() -> (w346:T9)
                  n152 = local read "MultiTrack"() -> (w345:cluster{"StartRow":i32, "EndRow":i32})
                  n153 = local read "Mode"() -> (w347:T8)
                  n154 = call "AndorSet.vi"("error in"=w349, "MultiTrack"=w345, "AcqSet"=w346, "Mode"=w347) -> ("error out"=w348:errorcluster, "SetStatus"=w343:bool, "SetOut"=w342:T11, "Timing"=w344:T10)  [unwired: 4 in]
                  n155 = local write "Timing"(w344) -> ()
                  n156 = local write "SetStatus"(w343) -> ()
                  n157 = local write "SetOut"(w342) -> ()
                }
                event "AndorSnap": Value Change {
                  n158 = event-data() -> ()  [unwired: 1 in, 6 out]
                  n159 = flat-sequence {
                    tunnel: [w357] -> w355
                    tunnel: w354 -> [w360]
                    tunnel: w355 -> [w372]
                    tunnel: [TRUE ("SaveStatus")] -> w353
                    tunnel: [w369] -> w352
                    frame #0 {
                      n160 = case shown="No Error" w360 {
                        tunnel: w360 -> [w363 w368]
                        tunnel: [w362 FALSE ("SaveStatus")] -> w359
                        tunnel: [w361 w368] -> w357
                        frame No Error {
                          n161 = local read "AcqSet"() -> (w365:T9)
                          n162 = Unbundle By Name(w365) -> ("KineticNum"=w364:i32)
                          n163 = call "AndorSaveasSif.vi"("error in"=w363, "KinNumber"=w364, "FilePath"="FilePath") -> ("error out"=w361:errorcluster, "SaveStatus"=w362:bool)  [unwired: 7 in]
                        }
                        frame Error {
                        }
                      }
                      n164 = Not(x=w359) -> (.not. x?=→"SaveStatus":bool)
                    }
                    frame #1 {
                      n165 = call <userlib>:"StartAcquisition.vi"("error in (no error)"=w372) -> ("error out"=w371:errorcluster)  [unwired: 1 in, 1 out]
                      n166 = while {
                        tunnel: w371 -> [w377]
                        tunnel: [w374] -> w369
                        stop <- w373 continue-if-true
                        n167 = call <userlib>:"GetStatus.vi"("error in (no error)"=w377) -> ("error out"=w374:errorcluster, "status"=w376:T20)  [unwired: 2 in, 1 out]
                        n168 = Equal?(x=w376, y=Error_Code_Enum_typedef."DRV_ACQUIRING") -> (x = y?=w373:bool)
                      }
                    }
                  }
                  n169 = local write "SaveStatus"(w353) -> ()
                }
                event "Exit": Value Change {
                  n170 = event-data() -> ()  [unwired: 1 in, 6 out]
                }
              }
            }
            frame "Exit" {
              n171 = local read "CoolerON"() -> (w389:T15)
              n172 = Unbundle By Name(w389) -> ("SetTemp"=w388:bool, "CoolerOn"=w387:bool)
              n173 = control-ref of="CurrentTemp"() -> (w386:refnum<vi>)
              n174 = control-ref of="ShutDown"() -> (w384:refnum<vi>)
              n175 = call "AndorShutdown.vi"("ShutDownRef"=w384, "CurrentTempRef"=w386, "error in"=w391, "CoolerON"=w387, "SetTemp"=w388) -> ("error out"=w390:errorcluster, "ShutDown"=w383:cluster{"CoolOff":bool, "ShutDown":bool}, "CurrentTemp"=w385:i32)  [unwired: 4 in]
              "ShutDown" <- w383
              n176 = local write "CurrentTemp"(w385) -> ()
              n177 = Unbundle By Name(w383) -> ("ShutDown"=w382:bool)  [unwired: 1 out]
            }
          }
        }
      }
    }
  }
